vi "Image Acquisition.vi"() -> ()   [LabVIEW 2017]
uses:
  Controls/FGV Actions.ctl
  Hardware/Thorlabs OCT/user.lib/SpectralRadar.llb/Processing Flag Selection.ctl
  Controls/Thorlabs Acq Status.ctl
  <extravilib>/ChannelInstances/Tag-bool/Read With Abort.vi
  <extravilib>/ChannelInstances/Tag-bool/Write With Abort.vi
  <extravilib>/ChannelInstances/Tag-bool/Instantiate.vi
  <extravilib>/ChannelInstances/Tag-bool/EndpointRead.vi
  <extravilib>/ChannelInstances/Tag-bool/Endpoint.vi
  Hardware/Thorlabs OCT/user.lib/SpectralRadar.llb/OCT Device.lvclass
  Hardware/Thorlabs OCT/user.lib/SpectralRadar.llb/Probe.lvclass
  Hardware/Thorlabs OCT/user.lib/SpectralRadar.llb/Raw Data.lvclass
  <extravilib>/ChannelInstances/Tag-bool.lvlib
  Hardware/Thorlabs OCT/user.lib/SpectralRadar.llb/Processing.lvclass
panel:
  in  "stop":bool
  in  "Aline Rate":u16(ring)=2 items=["76 KHz", "146 KHz", "76 KHz", "28 KHz", "10 KHz"]
  out "Probe":string="ProbeLKM10-LV"
  out "Scan Parameter":string="2048(Pix-Camera)-2048 (#Z Op)-0001(#Arpt)-05 (ArptExtra)-00400(#A)-060(BrtnExtra)-002(#Brpt)-400(#B)"
  in  "Objective":u16(ring)=1 items=["5X LKM05", "10X LKM10", "20X LKM20", "10X LSM02"]
  in  "# Cscan":i32=1
  out "Save Name":string="RAW-2048-0001-00400-002-400-"
  in  "Save Path":path=path "E:/Jiarui/1217test"
  in  "Shift (mm)":cluster{"Xshift (mm)":sgl, "Yshift (mm)":sgl}
  in  "ROI (mm)":cluster{"X (mm)":sgl, "Y (mm)":sgl}={"X (mm)"=1.0, "Y (mm)"=1.0}
  in  "# Rpt":cluster{"#ARpt":i32, "#BRpt":i32}={"#ARpt"=1, "#BRpt"=1}
  in  "# Scan":cluster{"#Ascan":i32, "#Bscan":i32}={"#Ascan"=400, "#Bscan"=400}
  out "Total Timel":dbl
  in  "?":bool
  out "DAQ B":i32
  out "Current C":i32=1
  out "iC Time":dbl
  out "Save B":i32
  out "subarray":u16[](graph)=[779, 535, 545, 559, 564, 576, 586, 586, 599, 600, 600, 608, 624, 627, 636, 655, 666, 671, 690, 721, 736, 766, 768, 791, 802, 844, 866, 892, 901, 936, 939, 965, 976, 1002, 999, 1028, 1042, 1057, 1052, 1073, 1078, 1096, 1119, 1142, 1139, 1161, 1162, 1198, 1211, 1251, 1267, 1284, 1300, 1328, 1340, 1383, 1407, 1446, 1449, 1495, 1487, 1527, 1545, 1593, 1632, 1661, 1689, 1714, 1719, 1758, 1794, 1829, 1860, 1893, 1895, 1916, 1933, 1963, 2002, 2054, 2054, 2100, 2100, 2118, 2133, 2189, 2227, 2283, 2289, 2331, 2342, 2370, 2402, 2455, 2490, 2532, 2515, 2540, 2495, 2518, 2534, 2579, 2585, 2581, 2537, 2525, 2522, 2531, 2573, 2618, 2645, 2674, 2690, 2706, 2763, 2822, 2922, 3017, 3017, 3078, 3101, 3135, 3125, 3184, 3232, 3280, 3291, 3306, 3245, 3239, 3219, 3269, 3273, 3310, 3279, 3208, 3158, 3157, 3177, 3205, 3221, 3222, 3234, 3208, 3197, 3240, 3266, 3314, 3322, 3356, 3305, 3291, 3258, 3251, 3282, 3333, 3316, 3314, 3293, 3264, 3242, 3285, 3308, 3373, 3353, 3341, 3293, 3281, 3242, 3249, 3307, 3310, 3341, 3370, 3343, 3289, 3294, 3334, 3369, 3415, 3422, 3364, 3302, 3335, 3346, 3360, 3443, 3429, 3398, 3334, 3312, 3305, 3326, 3353, 3303, 3275, 3220, 3190, 3111, 3123, 3107, 3137, 3087, 3068, 3058, 3063, 3051, 3088, 3123, 3178, 3236, 3286, 3314, 3316, 3389, 3353, 3386, 3359, 3360, 3370, 3347, 3367, 3360, 3356, 3355, 3323, 3329, 3277, 3230, 3213, 3126, 3129, 3115, 3105, 3074, 3075, 3041, 3014, 3039, 3082, 3118, 3119, 3154, 3142, 3098, 3082, 3105, 3145, 3139, 3205, 3146, 3148, 3103, 3124, 3127, 3153, 3111, 3112, 3105, 3118, 3098, 3070, 3047, 3052, 3047, 3077, 3089, 3060, 3036, 3039, 3067, 3106, 3154, 3146, 3162, 3165, 3157, 3177, 3182, 3202, 3228, 3198, 3201, 3154, 3141, 3166, 3228, 3242, 3234, 3258, 3199, 3208, 3173, 3153, 3115, 3138, 3147, 3124, 3057, 3049, 3003, 3003, 3042, 3054, 3046, 3061, 3039, 3056, 3046, 3113, 3157, 3176, 3155, 3173, 3176, 3216, 3236, 3260, 3240, 3235, 3235, 3244, 3197, 3134, 3071, 3085, 3109, 3098, 3060, 3027, 2988, 2980, 3002, 3046, 3033, 3030, 3009, 3010, 3015, 3027, 3024, 3031, 3061, 3106, 3084, 3087, 3015, 3039, 3018, 3020, 3026, 3011, 2986, 2981, 2975, 2987, 2965, 2915, 2882, 2887, 2882, 2891, 2856, 2849, 2832, 2854, 2914, 2910, 2883, 2896, 2869, 2925, 2934, 2928, 2950, 2940, 2957, 2998, 2998, 2937, 2909, 2905, 2932, 2964, 2956, 2967, 2924, 2950, 2966, 2913, 2874, 2868, 2869, 2866, 2833, 2797, 2761, 2785, 2805, 2814, 2813, 2792, 2757, 2788, 2837, 2866, 2876, 2850, 2878, 2905, 2889, 2864, 2829, 2871, 2931, 2967, 2921, 2876, 2862, 2873, 2854, 2826, 2744, 2753, 2776, 2782, 2746, 2712, 2697, 2699, 2724, 2708, 2678, 2705, 2709, 2730, 2753, 2751, 2722, 2771, 2807, 2802, 2762, 2779, 2769, 2825, 2785, 2789, 2754, 2781, 2781, 2792, 2747, 2744, 2718, 2729, 2719, 2692, 2673, 2653, 2653, 2702, 2648, 2655, 2659, 2700, 2725, 2699, 2654, 2673, 2704, 2734, 2733, 2725, 2729, 2787, 2756, 2748, 2750, 2774, 2788, 2788, 2761, 2745, 2742, 2770, 2726, 2716, 2679, 2696, 2751, 2725, 2662, 2667, 2670, 2681, 2667, 2641, 2629, 2669, 2653, 2657, 2622, 2665, 2680, 2696, 2666, 2682, 2682, 2709, 2704, 2717, 2706, 2757, 2759, 2752, 2718, 2721, 2751, 2769, 2722, 2654, 2653, 2663, 2620, 2611, 2563, 2580, 2605, 2597, 2551, 2570, 2607, 2605, 2553, 2549, 2555, 2599, 2617, 2613, 2625, 2662, 2696, 2657, 2629, 2655, 2684, 2702, 2640, 2638, 2644, 2672, 2622, 2593, 2576, 2601, 2603, 2602, 2551, 2551, 2555, 2513, 2487, 2489, 2504, 2520, 2492, 2486, 2499, 2525, 2498, 2490, 2507, 2549, 2542, 2545, 2513, 2542, 2569, 2580, 2520, 2543, 2571, 2585, 2543, 2508, 2527, 2524, 2495, 2468, 2467, 2512, 2487, 2432, 2434, 2434, 2421, 2411, 2370, 2403, 2405, 2377, 2359, 2378, 2396, 2420, 2389, 2403, 2405, 2443, 2414, 2421, 2431, 2463, 2427, 2427, 2414, 2446, 2399, 2398, 2377, 2393, 2398, 2379, 2331, 2341, 2328, 2306, 2262, 2260, 2281, 2283, 2238, 2230, 2251, 2266, 2238, 2227, 2266, 2310, 2271, 2279, 2321, 2335, 2300, 2294, 2299, 2333, 2304, 2298, 2298, 2321, 2321, 2288, 2272, 2278, 2267, 2232, 2239, 2257, 2231, 2184, 2169, 2194, 2186, 2151, 2127, 2171, 2193, 2173, 2159, 2210, 2187, 2176, 2177, 2194, 2207, 2202, 2197, 2224, 2231, 2225, 2230, 2244, 2259, 2205, 2198, 2203, 2192, 2156, 2140, 2182, 2164, 2149, 2114, 2130, 2136, 2137, 2101, 2118, 2106, 2109, 2083, 2112, 2122, 2140, 2114, 2145, 2158, 2150, 2123, 2162, 2191, 2168, 2157, 2188, 2196, 2198, 2178, 2198, 2196, 2184, 2168, 2193, 2186, 2170, 2133, 2188, 2163, 2132, 2121, 2132, 2138, 2131, 2128, 2132, 2102, 2114, 2124, 2141, 2158, 2159, 2170, 2210, 2179, 2183, 2189, 2222, 2210, 2227, 2238, 2265, 2245, 2236, 2246, 2253, 2218, 2232, 2248, 2237, 2227, 2230, 2191, 2196, 2182, 2192, 2198, 2204, 2192, 2213, 2204, 2171, 2173, 2214, 2212, 2238, 2242, 2271, 2267, 2260, 2284, 2294, 2298, 2324, 2325, 2353, 2348, 2333, 2334, 2327, 2308, 2315, 2334, 2326, 2309, 2304, 2295, 2279, 2259, 2276, 2251, 2286, 2260, 2262, 2234, 2246, 2254, 2287, 2293, 2298, 2304, 2321, 2329, 2336, 2359, 2364, 2341, 2354, 2361, 2372, 2375, 2384, 2392, 2380, 2344, 2358, 2351, 2356, 2346, 2341, 2362, 2328, 2308, 2310, 2276, 2291, 2299, 2300, 2295, 2288, 2275, 2300, 2280, 2301, 2290, 2317, 2330, 2336, 2334, 2346, 2333, 2336, 2345, 2344, 2373, 2373, 2360, 2369, 2359, 2352, 2317, 2341, 2328, 2324, 2311, 2314, 2302, 2296, 2274, 2271, 2261, 2247, 2247, 2271, 2228, 2233, 2236, 2257, 2230, 2229, 2264, 2249, 2242, 2245, 2266, 2290, 2262, 2271, 2303, 2295, 2275, 2282, 2294, 2298, 2266, 2285, 2275, 2260, 2223, 2236, 2231, 2209, 2203, 2209, 2202, 2178, 2135, 2156, 2133, 2139, 2123, 2134, 2147, 2150, 2140, 2126, 2139, 2162, 2145, 2161, 2187, 2186, 2154, 2181, 2180, 2169, 2149, 2172, 2182, 2176, 2157, 2175, 2162, 2143, 2123, 2128, 2119, 2102, 2090, 2112, 2088, 2084, 2075, 2052, 2050, 2033, 2033, 2041, 2064, 2065, 2036, 2075, 2056, 2012, 2005, 2065, 2071, 2071, 2073, 2088, 2078, 2066, 2056, 2078, 2052, 2051, 2089, 2084, 2084, 2052, 2027, 2020, 2000, 1998, 1986, 2013, 2009, 1989, 1966, 1973, 1942, 1941, 1922, 1961, 1954, 1976, 1966, 1968, 1922, 1952, 1954, 1950, 1966, 1973, 1968, 2010, 2006, 1996, 1977, 2016, 1998, 1979, 1988, 2034, 1999, 1997, 2004, 1993, 1962, 1976, 1953, 1965, 1979, 1977, 1951, 1954, 1946, 1915, 1896, 1927, 1928, 1911, 1940, 1960, 1941, 1938, 1933, 1939, 1936, 1961, 1965, 1981, 2017, 2000, 1975, 1986, 2007, 1983, 1978, 2025, 2004, 2006, 2025, 2015, 2014, 2006, 1969, 2000, 1992, 1992, 1962, 1992, 1999, 1968, 1948, 1985, 1973, 1967, 1972, 1992, 1978, 2016, 1996, 1999, 2014, 2027, 2011, 2039, 2088, 2088, 2077, 2118, 2105, 2097, 2099, 2123, 2107, 2142, 2126, 2107, 2138, 2125, 2080, 2120, 2106, 2102, 2085, 2110, 2082, 2103, 2082, 2074, 2059, 2093, 2065, 2059, 2085, 2101, 2063, 2121, 2126, 2108, 2139, 2144, 2130, 2174, 2208, 2169, 2217, 2261, 2239, 2245, 2259, 2238, 2248, 2260, 2261, 2273, 2292, 2292, 2271, 2331, 2280, 2231, 2253, 2263, 2244, 2258, 2276, 2237, 2260, 2256, 2207, 2268, 2257, 2250, 2278, 2306, 2268, 2332, 2282, 2301, 2349, 2351, 2322, 2395, 2418, 2395, 2410, 2454, 2410, 2441, 2416, 2409, 2447, 2454, 2418, 2477, 2486, 2424, 2429, 2424, 2383, 2435, 2420, 2388, 2437, 2466, 2405, 2414, 2429, 2375, 2419, 2427, 2394, 2468, 2527, 2462, 2517, 2553, 2492, 2534, 2549, 2549, 2644, 2649, 2602, 2703, 2677, 2629, 2648, 2657, 2622, 2700, 2659, 2661, 2750, 2670, 2617, 2681, 2615, 2586, 2624, 2597, 2609, 2652, 2569, 2608, 2612, 2560, 2546, 2584, 2564, 2624, 2640, 2602, 2667, 2709, 2633, 2686, 2679, 2673, 2746, 2768, 2756, 2830, 2839, 2790, 2825, 2801, 2793, 2862, 2788, 2821, 2884, 2819, 2821, 2863, 2773, 2836, 2788, 2726, 2797, 2807, 2747, 2826, 2825, 2742, 2817, 2765, 2742, 2814, 2795, 2790, 2857, 2836, 2837, 2876, 2821, 2901, 2927, 2858, 2933, 2989, 2917, 2974, 2977, 2921, 3042, 2914, 2930, 3009, 2920, 2939, 2972, 2911, 2925, 2948, 2836, 2911, 2903, 2838, 2953, 2837, 2831, 2905, 2829, 2844, 2900, 2823, 2877, 2902, 2832, 2931, 2931, 2888, 2974, 2975, 2985, 3045, 2987, 3018, 3097, 3045, 3099, 3123, 3087, 3146, 3130, 3074, 3152, 3101, 3133, 3112, 3056, 3148, 3111, 3030, 3120, 3038, 3033, 3077, 2939, 2972, 3027, 2925, 2997, 2964, 2922, 3033, 2952, 2917, 3041, 2941, 2987, 3028, 2976, 2984, 3085, 3034, 3131, 3085, 3110, 3172, 3106, 3220, 3081, 3005, 3166, 3156, 3173, 3227, 3076, 3151, 3144, 3060, 3163, 3104, 3080, 3142, 3031, 3056, 3102, 3031, 3053, 3020, 2985, 3066, 3082, 3072, 3099, 3028, 3132, 3112, 3100, 3153, 3127, 3208, 3227, 3191, 3306, 3221, 3222, 3276, 3219, 3210, 3298, 3226, 3283, 3286, 3250, 3270, 3147, 3193, 3158, 3118, 3164, 3117, 3124, 3190, 3050, 3101, 3046, 2982, 3056, 2979, 2976, 3057, 3021, 3061, 3067, 3013, 3078, 3040, 3058, 3067, 3078, 3190, 3121, 3171, 3254, 3210, 3293, 3200, 3198, 3281, 3218, 3250, 3278, 3262, 3329, 3284, 3285, 3248, 3171, 3263, 3160, 3152, 3244, 3121, 3253, 3192, 3111, 3177, 3076, 3105, 3141, 3098, 3136, 3094, 3138, 3141, 3098, 3170, 3084, 3093, 3149, 3091, 3194, 3179, 3105, 3190, 3144, 3192, 3177, 3130, 3177, 3160, 3230, 3202, 3154, 3231, 3177, 3117, 3165, 3059, 3136, 3078, 3090, 3082, 2991, 3095, 3027, 3021, 3055, 2918, 2935, 2974, 2991, 3055, 2986, 2999, 3059, 3061, 3089, 3003, 3034, 3004, 3048, 3096, 2988, 3121, 3072, 3160, 3230, 3156, 3199, 3217, 3175, 3046, 3001, 3247, 3234, 3195, 3222, 3130, 3169, 3135, 3082, 3089, 2939, 2871, 2947, 2990, 2995, 2897, 2925, 2872, 2862, 2897, 2882, 2921, 2779, 2769, 2899, 2840, 2911, 2848, 2912, 2920, 2916, 2949, 2706, 2847, 2871, 2933, 3031, 2937, 3018, 2972, 2982, 3067, 2965, 3011, 2795, 2878, 2904, 2844, 3000, 2926, 2897, 2795, 2644, 2874, 2823, 2766, 2805, 2681, 2452, 2574, 2827, 2810, 2788, 2889, 2830, 2904, 2873, 2879, 2868, 2821, 2946, 2898, 2931, 2946, 2867, 2913, 2915, 2916, 2573, 2517, 2873, 2840, 2947, 2877, 2861, 2749, 2761, 2765, 2717, 2802, 2751, 2753, 2776, 2713, 2742, 2705, 2742, 2659, 2557, 2610, 2551, 2601, 2562, 2604, 2566, 2510, 2632, 2435, 2550, 2626, 2570, 2623, 2585, 2561, 2375, 2649, 2684, 2689, 2765, 2692, 2738, 2698, 2716, 2721, 2710, 2764, 2541, 2689, 2753, 2740, 2730, 2645, 2689, 2567, 2617, 2361, 2475, 2648, 2596, 2622, 2541, 2582, 2487, 2504, 2497, 2421, 2441, 2439, 2512, 2478, 2486, 2505, 2413, 2467, 2399, 2437, 2422, 2440, 2483, 2461, 2512, 2442, 2475, 2442, 2414, 2432, 2379, 2433, 2401, 2456, 2417, 2365, 2337, 2357, 2352, 2285, 2295, 2270, 2268, 2284, 2246, 2283, 2234, 2294, 2232, 2212, 2186, 2149, 2174, 2128, 2128, 2183, 2223, 2221, 2218, 2225, 2191, 2245, 2195, 2247, 2216, 2267, 2274, 2270, 2257, 2222, 2218, 2186, 2234, 2244, 2255, 2246, 2228, 2273, 2207, 2242, 2217, 2195, 2122, 2097, 2111, 2058, 2027, 1847, 1824, 1908, 2019, 1981, 1906, 1969, 1938, 1951, 1934, 1941, 1897, 1921, 1928, 1926, 1950, 1895, 1822, 1800, 1710, 1724, 1834, 1842, 1894, 1952, 1938, 1978, 1914, 1956, 1895, 1838, 1883, 1934, 1941, 1944, 1942, 1934, 1936, 1905, 1892, 1864, 1800, 1781, 1850, 1861, 1844, 1880, 1824, 1845, 1803, 1854, 1808, 1801, 1767, 1777, 1825, 1822, 1845, 1832, 1851, 1832, 1837, 1832, 1830, 1828, 1826, 1809, 1705, 1791, 1774, 1798, 1744, 1769, 1798, 1797, 1785, 1781, 1764, 1744, 1771, 1750, 1743, 1702, 1709, 1699, 1651, 1642, 1644, 1649, 1646, 1648, 1623, 1640, 1588, 1597, 1564, 1586, 1567, 1566, 1579, 1592, 1588, 1579, 1603, 1572, 1572, 1550, 1527, 1534, 1543, 1444, 1511, 1602, 1608, 1622, 1594, 1592, 1590, 1605, 1583, 1611, 1589, 1602, 1602, 1600, 1591, 1593, 1592, 1549, 1542, 1527, 1522, 1499, 1414, 1462, 1514, 1506, 1487, 1442, 1419, 1476, 1431, 1450, 1439, 1462, 1412, 1344, 1390, 1388, 1395, 1430, 1404, 1415, 1387, 1392, 1391, 1399, 1394, 1408, 1416, 1400, 1393, 1368, 1376, 1341, 1348, 1340, 1343, 1354, 1362, 1339, 1337, 1339, 1320, 1302, 1239, 1213, 1245, 1272, 1265, 1275, 1242, 1274, 1256, 1254, 1225, 1205, 1132, 1195, 1205, 1228, 1222, 1230, 1221, 1227, 1221, 1228, 1231, 1217, 1211, 1214, 1224, 1225, 1233, 1254, 1259, 1252, 1257, 1244, 1232, 1220, 1215, 1198, 1184, 1202, 1193, 1215, 1215, 1207, 1173, 1175, 1143, 1142, 1117, 1120, 1082, 1072, 998, 1062, 1086, 1093, 1071, 1088, 1066, 1062, 1028, 1036, 1014, 1034, 1027, 1055, 1036, 1064, 1021, 1022, 1018, 1019, 978, 987, 971, 986, 993, 1009, 1028, 1034, 1009, 1013, 996, 989, 970, 971, 968, 965, 967, 977, 969, 974, 956, 934, 939, 915, 892, 910, 908, 906, 917, 928, 931, 925, 931, 923, 901, 908, 905, 898, 899, 893, 896, 906, 909, 923, 919, 903, 903, 901, 884, 883, 869, 882, 861, 874, 875, 880, 871, 865, 848, 848, 840, 841, 804, 800, 805, 822, 808, 799]
  # "ThorLabs TELESTO-3 OCT Imaging"
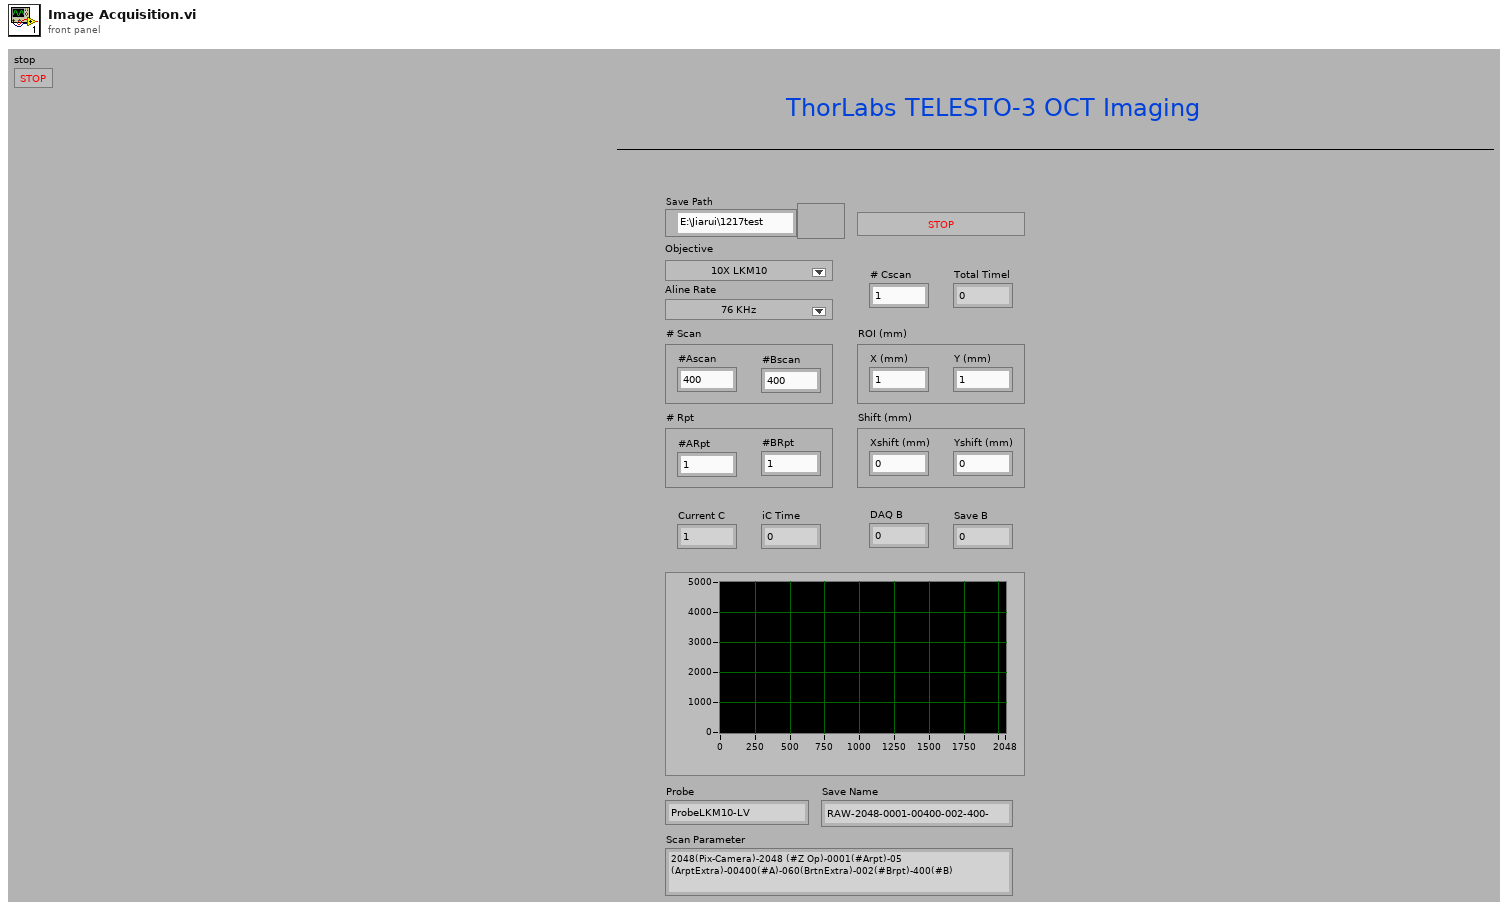
[diagram p1: front panel]
types:
  T1 = typedef "FGV Actions.ctl" = enum16{"Init", "Set", "Get", "Clear"}
  T2 = typedef "Processing.lvclass/Processing Flag Selection.ctl" = enum16{"Use Offset Errors", "Remove DC Spectrum", "Remove Advanced DC Spectrum", "Use Apodization", "Use Scan For Apodization", "Filter Undersampled Signals", "Use Dispersion Compensation", "Use Dechirp", "Use Extended Adjust", "Full Range Output", "Filter DC", "Autocorrelation Compensation", "DEFR", "Only Windowing", "Remove Fixed Pattern"}
  T3 = enum16{"FreeRunning", "TrigBoard_ExternalStart", "External_AScan"}
  T4 = enum16{"Asynchronous Continuous", "Asynchronous Finite", "Synchronous"}
  T5 = enum16{"open", "replace", "create", "open or create", "replace or create", "replace or create with confirmation"}
  T6 = enum16{"big-endian, network order", "native, host order", "little-endian"}
  T7 = typedef "Thorlabs Acq Status.ctl" = enum16{"Idle", "Image", "Translate"}
  T8 = typedef "Tag-bool.lvlib/))Channel.ctl" = refnum<queue>
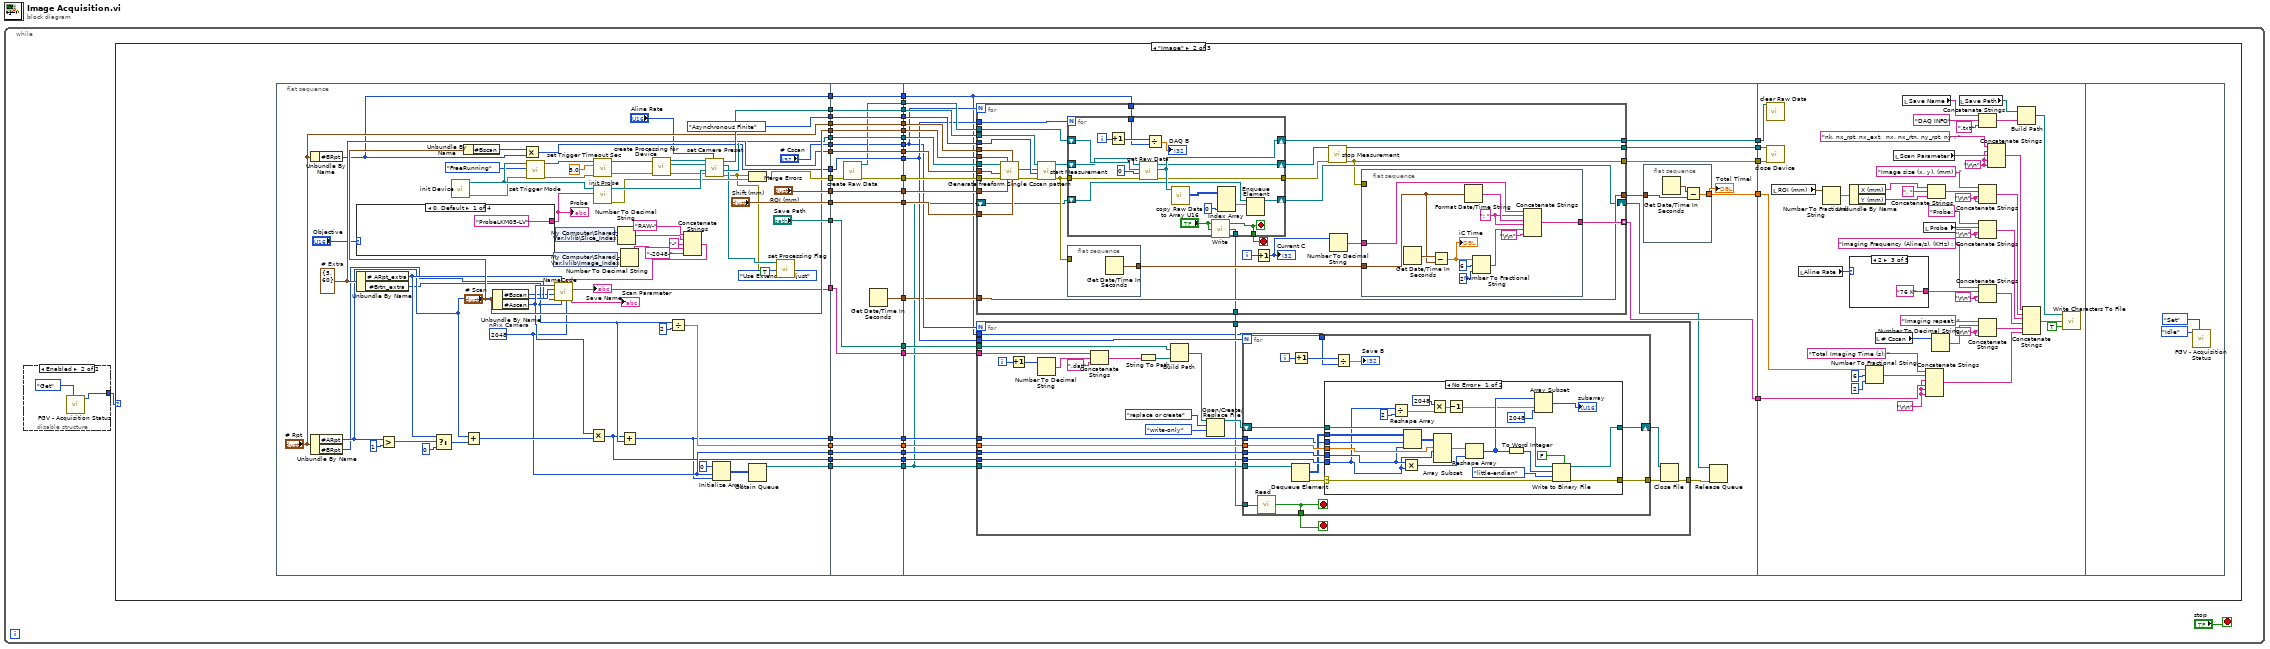
[diagram p0: block diagram]
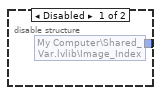
[diagram p2: hidden frame]
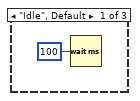
[diagram p3: hidden frame]
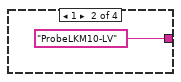
[diagram p4: hidden frame]
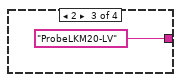
[diagram p5: hidden frame]
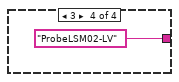
[diagram p6: hidden frame]
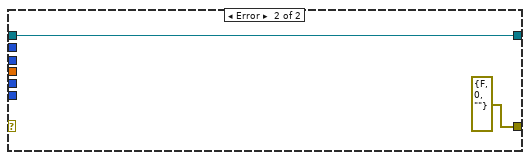
[diagram p7: hidden frame]
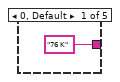
[diagram p8: hidden frame]
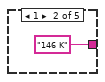
[diagram p9: hidden frame]
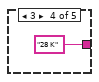
[diagram p10: hidden frame]
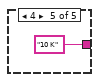
[diagram p11: hidden frame]
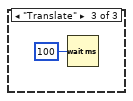
[diagram p12: hidden frame]
diagram:
  n1 = while {
    stop <- "stop" stop-if-true
    n2 = disable-structure shown="Enabled" {
      disable-tunnel: [w3 w4] -> w1
      frame Disabled {
        n3 = shared-variable "My Computer\\Shared_Var.lvlib\\Image_Index"() -> (w3:i16)  [unwired: 1 in, 1 out]
      }
      frame Enabled {
        n4 = call "FGV - Acquisition Status.vi"("Actions"=FGV_Actions."Get") -> ("Action [Out]"=w4:T7)  [unwired: 9 in, 1 out]
      }
    }
    n5 = case shown="\"Image\"" w1 {
      frame "Idle", Default {
        n6 = Wait (ms)(milliseconds to wait=u32 100) -> ()  [unwired: 1 out]
      }
      frame "Image" {
        n7 = flat-sequence {
          tunnel: [T4."Asynchronous Finite" ("Acquisition Type")] -> w51
          tunnel: [w112] -> w50
          tunnel: [w111] -> w49
          tunnel: [w79] -> w48
          tunnel: [w102] -> w47
          tunnel: ["Save Path"] -> w46
          tunnel: [w76] -> w45
          tunnel: [w84] -> w44
          tunnel: [w75] -> w43
          tunnel: ["Shift (mm)"] -> w42
          tunnel: ["# Rpt"] -> w41
          tunnel: ["ROI (mm)"] -> w40
          tunnel: ["# Scan"] -> w39
          tunnel: [w91] -> w38
          tunnel: [w90] -> w37
          tunnel: [w83] -> w36
          tunnel: ["# Cscan"] -> w35
          tunnel: [w74] -> w34
          tunnel: [w69] -> w33
          tunnel: w51 -> [w140]
          tunnel: w50 -> [w139]
          tunnel: w49 -> [w126]
          tunnel: w48 -> [w138]
          tunnel: w47 -> [w137]
          tunnel: w46 -> [w136]
          tunnel: w45 -> [w135]
          tunnel: w44 -> [w134]
          tunnel: w43 -> [w133]
          tunnel: w42 -> [w132]
          tunnel: w41 -> [w131]
          tunnel: w40 -> [w130]
          tunnel: w39 -> [w129]
          tunnel: w38 -> [w128]
          tunnel: w37 -> [w127]
          tunnel: [w140] -> w32
          tunnel: [w139] -> w31
          tunnel: [w138] -> w30
          tunnel: [w137] -> w29
          tunnel: [w136] -> w28
          tunnel: [w135] -> w27
          tunnel: [w134] -> w26
          tunnel: [w133] -> w25
          tunnel: [w132] -> w24
          tunnel: [w131] -> w23
          tunnel: [w130] -> w22
          tunnel: [w129] -> w21
          tunnel: [w128] -> w20
          tunnel: [w127] -> w19
          tunnel: [w125] -> w18
          tunnel: [w124] -> w17
          tunnel: [w123] -> w16
          tunnel: w36 -> [w123]
          tunnel: [w122] -> w15
          tunnel: w35 -> [w122]
          tunnel: [w121] -> w14
          tunnel: w34 -> [w121]
          tunnel: [w120] -> w13
          tunnel: [w119] -> w12
          tunnel: w33 -> [w119]
          tunnel: w32 -> [w170]
          tunnel: w31 -> [w169]
          tunnel: w30 -> [w153]
          tunnel: w29 -> [w141]
          tunnel: w28 -> [w158]
          tunnel: w27 -> [w157]
          tunnel: w26 -> [w155]
          tunnel: w25 -> [w156]
          tunnel: w24 -> [w168]
          tunnel: w23 -> [w167]
          tunnel: w22 -> [w166]
          tunnel: w21 -> [w165]
          tunnel: w20 -> [w164]
          tunnel: w19 -> [w163]
          tunnel: w18 -> [w162]
          tunnel: w17 -> [w161]
          tunnel: [w160] -> w11
          tunnel: [w159] -> w10
          tunnel: w16 -> [w154]
          tunnel: w15 -> [w152]
          tunnel: [w151] -> w9
          tunnel: w14 -> [w148]
          tunnel: w13 -> [w146]
          tunnel: [w145] -> w8
          tunnel: [w144] -> w7
          tunnel: w12 -> [w142]
          tunnel: w11 -> [w344]
          tunnel: w10 -> [w345]
          tunnel: w9 -> [w322]
          tunnel: w8 -> [w319]
          tunnel: w7 -> [w308]
          frame #0 {
            w91 = cluster{"# ARpt_extra":i32, "#Brtn_extra":i32} {"# ARpt_extra"=5, "#Brtn_extra"=60}  # # Extra
            w84 = 2048  # nPix Camera
            n8 = Unbundle By Name("# Rpt") -> ("#BRpt"=w69:i32)
            n9 = Unbundle By Name("# Rpt") -> ("#ARpt"=w86:i32, "#BRpt"=w78:i32)
            n10 = case shown="0, Default" "Objective" {
              tunnel: ["ProbeLKM05-LV" ("Probe") "ProbeLKM10-LV" ("Probe") "ProbeLKM20-LV" ("Probe") "ProbeLSM02-LV" ("Probe")] -> w72
              frame 0, Default {
              }
              frame 1 {
              }
              frame 2 {
              }
              frame 3 {
              }
            }
            "Probe" <- w72
            n11 = Unbundle By Name(w91) -> ("# ARpt_extra"=w88:i32, "#Brtn_extra"=w85:i32)
            n12 = Greater?(x=w86, y=1) -> (0:w98:bool)
            n13 = Select(t=w88, s=w98, f=0) -> (s? t:f=w96:i32)
            n14 = call "init Device.vi"() -> ("error out"=w109:errorcluster, "OCTDevice"=w110:refnum<class "OCT Device.lvclass">)  [unwired: 6 in]
            n15 = Unbundle By Name("# Scan") -> ("#Bscan"=w80:i32)
            n16 = Add(x=w86, y=w96) -> (x+y=w89:i32)
            n17 = Unbundle By Name("# Scan") -> ("#Bscan"=w77:i32, "#Ascan"=w87:i32)
            n18 = Multiply(x=w80, y=w69) -> (x*y=w79:i32)
            n19 = call "set Trigger Mode.vi"("error in (no error)"=w109, "Trigger Type"=T3."FreeRunning", "OCTDevice in"=w110) -> ("error out"=w106:errorcluster, "OCTDevice out"=w107:refnum<class "OCT Device.lvclass">)  [unwired: 3 in]
            n20 = shared-variable "My Computer\\Shared_Var.lvlib\\Image_Index"() -> (w54:i16)  [unwired: 1 in, 1 out]
            n21 = shared-variable "My Computer\\Shared_Var.lvlib\\Slice_Index"() -> (w58:i16)  [unwired: 1 in, 1 out]
            n22 = Multiply(x=w87, y=w89) -> (x*y=w75:i32)
            n23 = call "set Trigger Timeout Sec.vi"("error in (no error)"=w106, "Trigger Timeout"=5.0, "OCTDevice in"=w107) -> ("error out"=w64:errorcluster, "OCTDevice out"=w68:refnum<class "OCT Device.lvclass">)  [unwired: 3 in]
            n24 = call "init Probe.vi"("Probe"=w72, "OCT Device"=w110) -> ("error out"=w95:errorcluster, "GalvoControl"=w114:refnum<class "Probe.lvclass">)  [unwired: 4 in]
            n25 = Number To Decimal String(number=w58) -> (decimal integer string=w57:string)  [unwired: 1 in]
            n26 = Number To Decimal String(number=w54) -> (decimal integer string=w53:string)  [unwired: 1 in]
            n27 = Add(x=w75, y=w85) -> (x+y=w74:i32)
            n28 = call "create Processing for Device.vi"("error in (no error)"=w64, "OCTDevice"=w68) -> ("error out"=w65:errorcluster, "Processing"=w66:refnum<class "Processing.lvclass">, "OCTDevice"=w67:refnum<class "OCT Device.lvclass">)  [unwired: 3 in]
            n29 = Divide(x=w85, y=2) -> (x/y=w76:dbl)
            n30 = Concatenate Strings("RAW-" ("Name0"), w57, "-" ("string"), w53, "-2048-" ("string")) -> (w55:string)
            n31 = call "NameCode.vi"("# Z"=w84, "Name0"=w55, "# BRtn extra"=w85, "# ARpt extra"=w88, "# B rpt"=w78, "# B scan"=w77, "# A rpt"=w86, "# Aline"=w87) -> ("Scan Parameter"=→"Scan Parameter":string, "Name Code"=w83:string)  [unwired: 2 in]
            "Save Name" <- w83
            n32 = call "set Camera Preset.vi"("Numeric"="Aline Rate", "error in (no error)"=w65, "Probe"=w114, "Processing"=w66, "OCTDevice"=w67) -> ("error out"=w60:errorcluster, "Probe 2"=w90:refnum<class "Probe.lvclass">, "Processing"=w61:refnum<class "Processing.lvclass">, "OCTDevice out"=w112:refnum<class "OCT Device.lvclass">)  [unwired: 1 in]
            n33 = Initialize Array(u16 0 ("element"), w84, w74) -> (w104:u16[][])
            n34 = Merge Errors(w60, w95) -> (w111:errorcluster)
            n35 = Obtain Queue(element data type=w104) -> (queue out=w102:refnum<queue>)  [unwired: 3 in, 3 out]
            n36 = call "set Processing Flag.vi"("error in (no error)"=w60, "Flag"=TRUE, "Processing Flag Selection"=Processing_Flag_Selection."Use Extended Adjust", "Processing"=w61) -> ()  [unwired: 2 in, 2 out]
          }
          frame #1 {
            n37 = call "create Raw Data.vi"("error in (no error)"=w126) -> ("error out"=w125:errorcluster, "Raw Data"=w124:refnum<class "Raw Data.lvclass">)  [unwired: 5 in]
            n38 = Get Date/Time In Seconds() -> (seconds since 1Jan1904=w120:timestamp)
          }
          frame #2 {
            n39 = for {
              N: w152 -> [_]
              tunnel: w170 -> [w204]
              tunnel: w168 -> [w202]
              tunnel: w167 -> [w201]
              tunnel: w166 -> [w200]
              tunnel: w165 -> [w199]
              tunnel: w164 -> [w198]
              tunnel: w163 -> [w197]
              tunnel: w153 -> [w185]
              tunnel: w161 -> [w196]
              tunnel: [w195] -> w160
              tunnel: w169 -> [w203]
              tunnel: [w194] -> w159
              tunnel: w162 -> [w193]
              tunnel: [w192] -> w151 mode=indexing
              shift-right: [w178] -> w149
              shift-left: w141 -> [w184]
              tunnel: [w181] -> w147
              tunnel: w146 -> [w181]
              tunnel: [w177] -> w144
              tunnel: [w176] -> w143
              tunnel: w142 -> [w175]
              i -> [w186]
              stop <- w174 stop-if-true
              n40 = call "Generate freeform Single Cscan pattern.vi"("Shift (mm)"=w202, "# Rpt"=w201, "ROI (mm)"=w200, "# Scan"=w199, "error in (no error)"=w193, "# Extra"=w198, "Probe"=w197) -> ("error out"=w188:errorcluster, "Scan Pattern"=w189:refnum<class "Scan Pattern.lvclass">)  [unwired: 1 in, 2 out]
              n41 = call "start Measurement.vi"("error in (no error)"=w188, "Acquisition Type"=w204, "Scan Pattern"=w189, "OCTDevice"=w203) -> ("error out"=w187:errorcluster, "OCTDevice"=w191:refnum<class "OCT Device.lvclass">)  [unwired: 1 in, 1 out]
              n42 = for {
                N: w185 -> [_]
                tunnel: w187 -> [w218]
                shift-right: [w221] -> w195
                shift-left: w196 -> [w222]
                shift-right: [w219] -> w190
                shift-left: w191 -> [w220]
                tunnel: [w209] -> w183
                shift-right: [w208] -> w178
                shift-left: w184 -> [w214]
                tunnel: [w207] -> w176
                tunnel: w175 -> [w206]
                tunnel: ["?"] -> w174
                i -> [w212]
                stop <- "?" stop-if-true
                n43 = Increment(x=w212) -> (x+1=w211:i32)
                n44 = call "get Raw Data.vi"("error in (no error)"=w218, "Camera Index"=0, "RawData in"=w222, "OCTDevice in"=w220) -> ("error out"=w209:errorcluster, "RawData out"=w221:refnum<class "Raw Data.lvclass">, "OCTDevice out"=w219:refnum<class "OCT Device.lvclass">)  [unwired: 1 in]
                n45 = Divide(x=w211, y=w206) -> (x/y=→"DAQ B":dbl)
                n46 = call "copy Raw Data to Array U16.vi"("Data in"=w221) -> ("Data Content"=w216:u16[][][])  [unwired: 4 in, 2 out]
                n47 = call <extravilib>:"Write.vi"("element"="?") -> ("channel"=w207:T8)  [unwired: 1 out]
                n48 = Index Array(array=w216, index (dim 2)=0 ("index (page)")) -> (element=w213:u16[][])  [unwired: 2 in]
                n49 = Enqueue Element(queue=w214, element=w213) -> (queue out=w208:refnum<queue>)  [unwired: 1 in, 3 out]
              }
              n50 = flat-sequence {
                tunnel: w187 -> [_]
                tunnel: [w223] -> w182
                frame #0 {
                  n51 = Get Date/Time In Seconds() -> (seconds since 1Jan1904=w223:timestamp)
                }
              }
              n52 = Increment(x=w186) -> (x+1=w180:i32)
              "Current C" <- w180
              n53 = call "stop Measurement.vi"("error in (no error)"=w183, "OCTDevice"=w190) -> ("error out"=w177:errorcluster, "OCTDevice"=w194:refnum<class "OCT Device.lvclass">)  [unwired: 4 in]
              n54 = Number To Decimal String(number=w180) -> (decimal integer string=w179:string)  [unwired: 1 in]
              n55 = flat-sequence {
                tunnel: w177 -> [_]
                tunnel: [w230] -> w192
                tunnel: w182 -> [w226]
                tunnel: w179 -> [w224]
                frame #0 {
                  w225 = ": " ("string")
                  n56 = Get Date/Time In Seconds() -> (seconds since 1Jan1904=w234:timestamp)
                  n57 = Subtract(x=w234, y=w226) -> (x-y=w231:dbl)
                  "iC Time" <- w231
                  n58 = Format Date/Time String(seconds (now)=w226) -> (date/time string=w229:string)  [unwired: 2 in]
                  n59 = Number To Fractional String(number=w231, width (-)=i16 6, precision (6)=i16 2) -> (F-format string=w228:string)  [unwired: 1 in]
                  n60 = Concatenate Strings(w224, w225, w229, w225, w228, "\r\n") -> (w230:string)
                }
              }
            }
            n61 = for {
              N: w152 -> [_]
              tunnel: w141 -> [w258]
              tunnel: w154 -> [w249]
              tunnel: [w246] -> w150
              tunnel: w158 -> [w245]
              tunnel: w157 -> [w244]
              tunnel: w156 -> [w243]
              tunnel: w155 -> [w242]
              tunnel: w153 -> [w241]
              tunnel: w148 -> [w240]
              tunnel: w143 -> [w237]
              tunnel: w142 -> [w236]
              i -> [w239]
              stop <- w235 stop-if-true
              n62 = Increment(x=w239) -> (x+1=w238:i32)
              n63 = Number To Decimal String(number=w238) -> (decimal integer string=w251:string)  [unwired: 1 in]
              n64 = Concatenate Strings(w249, w251, ".dat" ("string")) -> (w253:string)
              n65 = String To Path(string=w253) -> (path=w254:path)
              n66 = Build Path(base path=w245, name or relative path=w254) -> (appended path=w255:path)
              n67 = Open/Create/Replace File(file path (use dialog)=w255, operation (0:open)=T5."replace or create", access (0:read/write)=enum16{"read/write", "read-only", "write-only"}."write-only") -> (refnum out=w250:refnum<file>)  [unwired: 3 in, 2 out]
              n68 = for {
                N: w241 -> [_]
                tunnel: w258 -> [w274]
                tunnel: [w271] -> w247
                tunnel: w244 -> [w270]
                tunnel: w243 -> [w269]
                tunnel: w242 -> [w267]
                shift-right: [w272] -> w248
                shift-left: w250 -> [w273]
                tunnel: w240 -> [w265]
                tunnel: w237 -> [w261]
                tunnel: w236 -> [w260]
                tunnel: [w259] -> w235
                i -> [w262]
                stop <- w259 stop-if-true
                n69 = call <extravilib>:"Read.vi"("channel"=w261) -> ("element"=w259:bool)  [unwired: 1 in, 1 out]
                n70 = Dequeue Element(queue=w274) -> (element=w266:u16[][], error out=w268:errorcluster)  [unwired: 1 in, 3 out]
                n71 = Increment(x=w262) -> (x+1=w264:i32)
                n72 = case shown="No Error" w268 {
                  selector: w268 -> [w294 _]
                  tunnel: w266 -> [w282 _]
                  tunnel: w273 -> [w295 w299]
                  tunnel: [w293 w299] -> w272
                  tunnel: [w292 errorcluster {"status"=FALSE, "code"=0, "source"=""} ("error out")] -> w271
                  tunnel: w270 -> [w287 _]
                  tunnel: w269 -> [w280 _]
                  tunnel: w267 -> [w285 _]
                  tunnel: w265 -> [w290 _]
                  frame No Error {
                    n73 = Divide(x=w280, y=2) -> (x/y=w278:dbl)
                    n74 = Multiply(x=w285, y=w280) -> (x*y=w286:i32)
                    n75 = Reshape Array(w282, w290, w285) -> (w289:u16[][])
                    n76 = Multiply(x=2048 ("length"), y=w278) -> (x*y=w276:dbl)
                    n77 = Array Subset(array=w289, index (row)=w287, length (row)=w280) -> (w288:u16[][])  [unwired: 2 in]
                    n78 = Decrement(x=w276) -> (x-1=w275:dbl)
                    n79 = Reshape Array(w288, w286) -> (w281:u16[])
                    n80 = To Word Integer(number=w281) -> (16bit integer=w291:i16[])
                    n81 = Array Subset(array=w281, index=w275, length=2048) -> (→"subarray":u16[])
                    n82 = Write to Binary File(file (use dialog)=w295, data=w291, error in=w294, 5:FALSE ("prepend array or string size? (T)"), 9:T6."little-endian" ("byte order (0:big-endian, network order)")) -> (refnum out=w293:refnum<file>, error out=w292:errorcluster)  [unwired: 1 in, 1 out]
                  }
                  frame Error {
                  }
                }
                n83 = Divide(x=w264, y=w260) -> (x/y=→"Save B":dbl)
              }
              n84 = Close File(refnum=w248, error in=w247) -> (error out=w246:errorcluster)  [unwired: 1 out]
            }
            n85 = flat-sequence {
              tunnel: [w172] -> w145
              tunnel: w147 -> [w171]
              frame #0 {
                n86 = Get Date/Time In Seconds() -> (seconds since 1Jan1904=w173:timestamp)
                n87 = Subtract(x=w173, y=w171) -> (x-y=w172:dbl)
              }
            }
            n88 = Release Queue(queue=w149, error in (no error)=w150) -> ()  [unwired: 1 in, 3 out]
            "Total Timel" <- w145
          }
          frame #3 {
            w306 = "\r\n"
            w314 = "\r\n"
            w316 = "\r\n"
            w333 = "\r\n"
            w334 = "\r\n"
            w302 = "\r\n"
            n89 = call "clear Raw Data.vi"("Raw Data"=w344) -> ()  [unwired: 6 in, 1 out]
            n90 = call "close Device.vi"("error in (no error)"=w308, "OCTDevice"=w345) -> ()  [unwired: 5 in, 1 out]
            n91 = local read "ROI (mm)"() -> (w301:cluster{"X (mm)":sgl, "Y (mm)":sgl})
            n92 = local read "Aline Rate"() -> (w307:u16)
            n93 = Number To Fractional String(number=w301) -> (F-format string=w300:cluster{"X (mm)":string, "Y (mm)":string})  [unwired: 3 in]
            n94 = Unbundle By Name(w300) -> ("X (mm)"=w339:string, "Y (mm)"=w340:string)
            n95 = case shown="2" w307 {
              tunnel: ["76 K" "146 K" "76 K" "28 K" "10 K"] -> w305
              frame 0, Default {
              }
              frame 1 {
              }
              frame 2 {
              }
              frame 3 {
              }
              frame 4 {
              }
            }
            n96 = Number To Fractional String(number=w319, width (-)=i16 6, precision (6)=i16 2) -> (F-format string=w317:string)  [unwired: 1 in]
            n97 = local read "# Cscan"() -> (w323:i32)
            n98 = local read "Scan Parameter"() -> (w315:string)
            n99 = local read "Save Name"() -> (w326:string)
            n100 = local read "Probe"() -> (w312:string)
            n101 = Concatenate Strings("Total Imaging Time (s): " ("string"), w317, w316, w322, w316, w316) -> (w310:string)
            n102 = Concatenate Strings(w339, ", " ("string"), w340) -> (w341:string)
            n103 = Number To Decimal String(number=w323) -> (decimal integer string=w335:string)  [unwired: 1 in]
            n104 = local read "Save Path"() -> (w327:path)
            n105 = Concatenate Strings("Image size (x, y), (mm) : " ("string"), w341, w334, w334) -> (w331:string)
            n106 = Concatenate Strings("Probe: " ("string"), w312, w314, w314) -> (w311:string)
            n107 = Concatenate Strings("Imaging Frequency (Aline/s), (KHz) : " ("string"), w305, w306, w306) -> (w303:string)
            n108 = Concatenate Strings("Imaging repeat: " ("string"), w335, w333, w333) -> (w309:string)
            n109 = Concatenate Strings(w326, "DAQ INFO" ("string"), ".txt" ("string")) -> (w343:string)
            n110 = Concatenate Strings("nk, nx_rpt, nx_ext,  nx, nx_rtn, ny_rpt, ny : " ("string"), w302, w315, w302, w302) -> (w332:string)
            n111 = Build Path(base path=w327, name or relative path=w343) -> (appended path=w329:path)
            n112 = Concatenate Strings(w332, w331, w311, w303, w309, w310) -> (w330:string)
            n113 = call <vilib>:"Write Characters To File.vi"("append to file? (new file:F)"=TRUE, "character string"=w330, "file path (dialog if empty)"=w329) -> ()  [unwired: 2 in, 1 out]
          }
          frame #4 {
            n114 = call "FGV - Acquisition Status.vi"("Actions"=FGV_Actions."Set", "Action"=Thorlabs_Acq_Status."Idle") -> ()  [unwired: 8 in, 2 out]
          }
        }
      }
      frame "Translate" {
        n115 = Wait (ms)(milliseconds to wait=u32 100) -> ()  [unwired: 1 out]
      }
    }
  }
